vi "Time Zone String.vi"(11 "Time Zone":T1(ring)) -> (3 "Time Zone String":string)   [LabVIEW 2015]
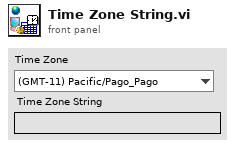
[diagram p1: front panel]
types:
  T1 = enum16{"(GMT-11) Pacific/Pago_Pago", "(GMT-10) Pacific/Johnston", "(GMT-9) America/Anchorage", "(GMT-6) America/Chicago", "(GMT-5) America/Lima", "(GMT-4) America/Grenada", "(GMT-3) Atlantic/Stanley", "(GMT-2) Atlantic/South_Georgia", "(GMT-1) Atlantic/Azores", "(GMT) Europe/London", "(GMT+1) Europe/Amsterdam", "(GMT+2) Africa/Blantyre", "(GMT+3) Africa/Djibouti", "(GMT+4) Asia/Baku", "(GMT+5) Asia/Dushanbe", "(GMT+5.30) Asia/Colombo", "(GMT+6) Asia/Dhaka", "(GMT+6:30) Indian/Cocos", "(GMT+7) Asia/Krasnoyarsk", "(GMT+8) Asia/Taipei", "(GMT+9) Pacific/Tongatapu", "(GMT+9:30) Australia/North", "(GMT+10) Australia/Lindeman", "(GMT+10:30) Australia/Yancowinna", "(GMT+11) Australia/Canberra", "(GMT+12) Asia/Kamchatka", "(GMT+13) Pacific/Auckland", "(GMT+14) Pacific/Apia"}
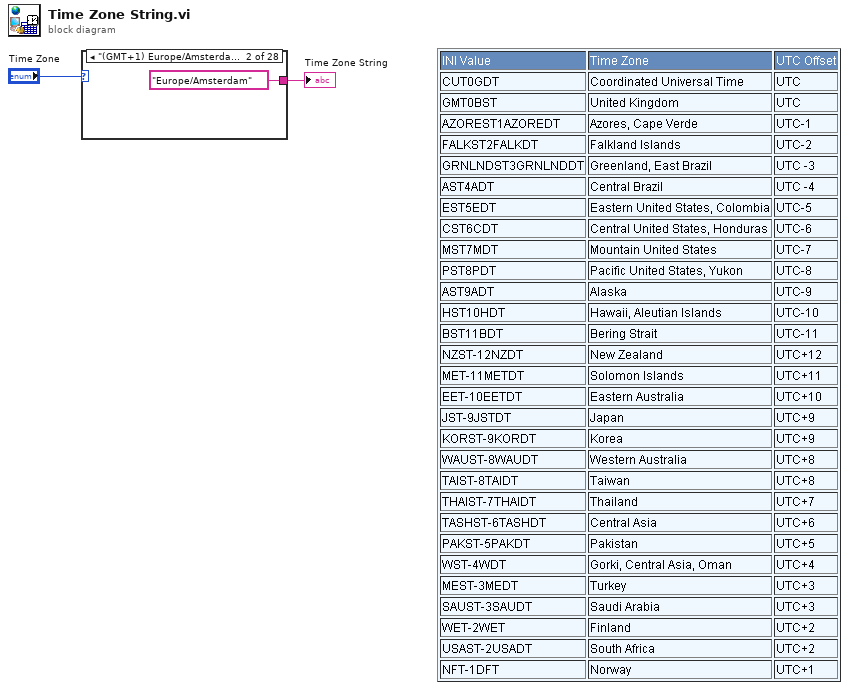
[diagram p0: block diagram]
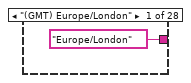
[diagram p2: hidden frame]
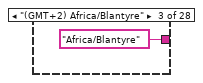
[diagram p3: hidden frame]
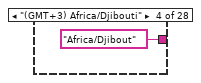
[diagram p4: hidden frame]
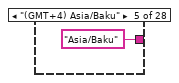
[diagram p5: hidden frame]
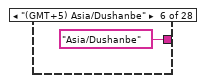
[diagram p6: hidden frame]
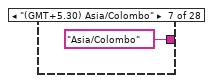
[diagram p7: hidden frame]
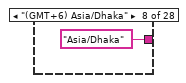
[diagram p8: hidden frame]
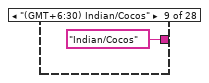
[diagram p9: hidden frame]
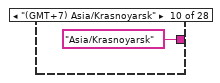
[diagram p10: hidden frame]
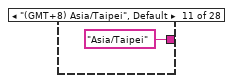
[diagram p11: hidden frame]
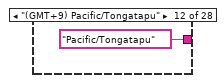
[diagram p12: hidden frame]
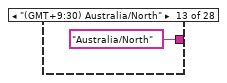
[diagram p13: hidden frame]
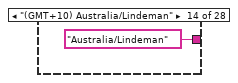
[diagram p14: hidden frame]
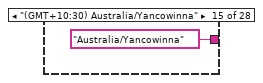
[diagram p15: hidden frame]
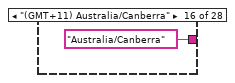
[diagram p16: hidden frame]
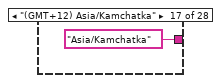
[diagram p17: hidden frame]
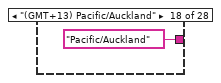
[diagram p18: hidden frame]
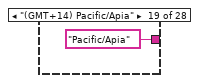
[diagram p19: hidden frame]
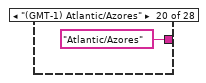
[diagram p20: hidden frame]
diagram:
  n1 = case shown="\"(GMT+1) Europe/Amsterdam\"" "Time Zone" {
    tunnel: ["Europe/London" "Europe/Amsterdam" "Africa/Blantyre" "Africa/Djibout" "Asia/Baku" "Asia/Dushanbe" "Asia/Colombo" "Asia/Dhaka" "Indian/Cocos" "Asia/Krasnoyarsk" "Asia/Taipei" "Pacific/Tongatapu" "Australia/North" "Australia/Lindeman" "Australia/Yancowinna" "Australia/Canberra" "Asia/Kamchatka" "Pacific/Auckland" "Pacific/Apia" "Atlantic/Azores" "Atlantic/South_Georgia" "Atlantic/Stanley" "America/Grenada" "America/Lima" "America/Chicago" "America/Anchorage" "Pacific/Johnston" "Pacific/Pago_Pago"] -> w1
    frame "(GMT) Europe/London" {
    }
    frame "(GMT+1) Europe/Amsterdam" {
    }
    frame "(GMT+2) Africa/Blantyre" {
    }
    frame "(GMT+3) Africa/Djibouti" {
    }
    frame "(GMT+4) Asia/Baku" {
    }
    frame "(GMT+5) Asia/Dushanbe" {
    }
    frame "(GMT+5.30) Asia/Colombo" {
    }
    frame "(GMT+6) Asia/Dhaka" {
    }
    frame "(GMT+6:30) Indian/Cocos" {
    }
    frame "(GMT+7) Asia/Krasnoyarsk" {
    }
    frame "(GMT+8) Asia/Taipei", Default {
    }
    frame "(GMT+9) Pacific/Tongatapu" {
    }
    frame "(GMT+9:30) Australia/North" {
    }
    frame "(GMT+10) Australia/Lindeman" {
    }
    frame "(GMT+10:30) Australia/Yancowinna" {
    }
    frame "(GMT+11) Australia/Canberra" {
    }
    frame "(GMT+12) Asia/Kamchatka" {
    }
    frame "(GMT+13) Pacific/Auckland" {
    }
    frame "(GMT+14) Pacific/Apia" {
    }
    frame "(GMT-1) Atlantic/Azores" {
    }
    frame "(GMT-2) Atlantic/South_Georgia" {
    }
    frame "(GMT-3) Atlantic/Stanley" {
    }
    frame "(GMT-4) America/Grenada" {
    }
    frame "(GMT-5) America/Lima" {
    }
    frame "(GMT-6) America/Chicago" {
    }
    frame "(GMT-9) America/Anchorage" {
    }
    frame "(GMT-10) Pacific/Johnston" {
    }
    frame "(GMT-11) Pacific/Pago_Pago" {
    }
  }
  "Time Zone String" <- w1
